vi "Acceleration.vi"(2 "Y Input":dbl, 3 "X Input":dbl) -> (0 "Y Output":dbl format="%.2f", 1 "X Output":dbl format="%.2f")   [LabVIEW 2013]
uses:
  <vilib>/addons/control/pid/pid.llb/PID Lead-Lag (DBL).vi
  <vilib>/addons/control/pid/NI_PID_pid.lvlib
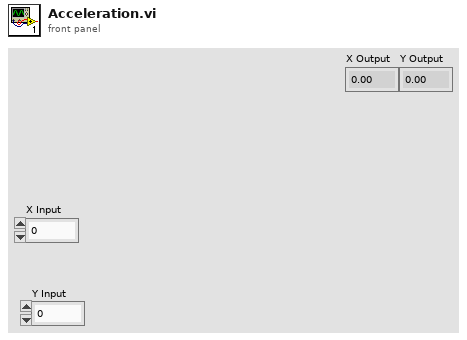
[diagram p1: front panel]
types:
  T1 = cluster{"gain":dbl, "lag time (min)":dbl, "lead time (min)":dbl}
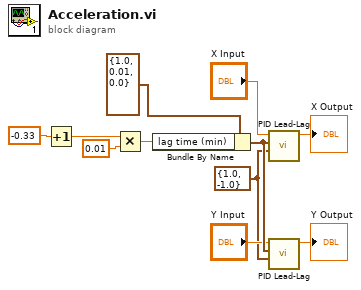
[diagram p0: block diagram]
diagram:
  w3 = cluster{"output high":dbl, "output low":dbl} {"output high"=1.0, "output low"=-1.0} ("output range")
  n1 = Increment(x=-0.33) -> (x+1=w7:dbl)
  n2 = Multiply(x=w7, y=0.01) -> (x*y=w10:dbl)
  n3 = Bundle By Name(cluster=T1 {"gain"=1.0, "lag time (min)"=0.01, "lead time (min)"=0.0} ("tuning parameters"), "lag time (min)"=w10) -> (w11:T1)
  n4 = call-poly <vilib>:"PID Lead-Lag.vi"("output range"=w3, "tuning parameters"=w11, "input"="X Input") -> ("output"=→"X Output":dbl)  [unwired: 3 in, 3 out]
  n5 = call-poly <vilib>:"PID Lead-Lag.vi"("output range"=w3, "tuning parameters"=w11, "input"="Y Input") -> ("output"=→"Y Output":dbl)  [unwired: 3 in, 3 out]
